vi "AK-LNI Befehl und Antwort_ALT.vi"(7 "Kanalnummer (0)":u8 max=99 step=1, 8 "Fehler (Eingang)":errorcluster, 9 "Sendedaten":string[](array[string]), 10 "Befehl (4 Zeichen)":string, 11 "VISA resource name":refnum<visa-resource-name>) -> (0 "Fehler (Ausgang)":errorcluster, 1 "ES (Error Status)":string, 2 "Empfangsdaten":string[](array[string]), 3 "VISA resource name out":refnum<visa-resource-name>, 4 "Daten":string, 5 "Befehl (Antwort)":string)   [LabVIEW 2020, in "Linearisierung v2.lvlib" / "Gasteiler.lvlib" / "AK Komm Gasteiler.lvlib" / "Alter Gasteiler.lvlib"]
doc: "Vollständige Gerätekommunikation für Inbetriebnahme und als Muster für spezielle Befehle. Sendet ein vollständiges Befehls-Telegramm und liefert die Geräteantwort als 1D-Array aus Strings \"Empfangsdaten\", in dem die einzelnen Argumente getrennt verfügbar sind.\n\n\"Befehl\": immer vier ASCII-Zeichen (Großbuchstaben)\n\n\"Daten\": 1D-Array aus ASCII-Strings nach Vorgabe des Befehls."
uses:
  Alter Gasteiler.lvlib
  AK Komm Gasteiler.lvlib
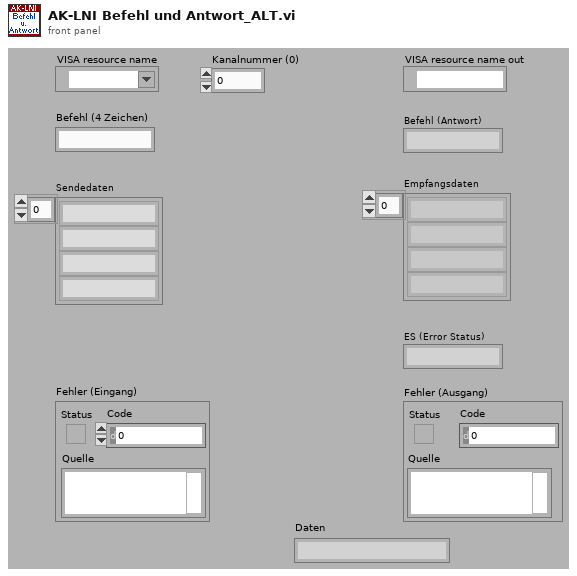
[diagram p1: front panel]
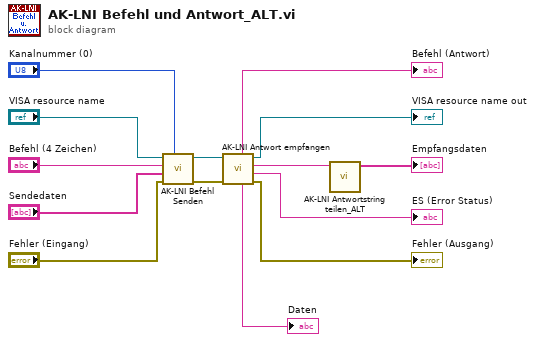
[diagram p0: block diagram]
diagram:
  n1 = call "AK-LNI Befehl Senden.vi"("Kanalnummer (K0)"="Kanalnummer (0)", "Fehler (Eingang)"="Fehler (Eingang)", "Daten"="Sendedaten", "Befehl (4 Zeichen)"="Befehl (4 Zeichen)", "VISA resource name"="VISA resource name") -> ("Fehler (Ausgang)"=w11:errorcluster, "VISA resource name out"=w13:refnum<visa-resource-name>)  [unwired: 5 in]
  n2 = call "AK-LNI Antwort empfangen.vi"("Fehler (Eingang)"=w11, "VISA resource name"=w13) -> ("Fehler (Ausgang)"=→"Fehler (Ausgang)":errorcluster, "ES (Error Status)"=→"ES (Error Status)":string, "Daten"=w4:string, "VISA resource name out"=→"VISA resource name out":refnum<visa-resource-name>, "Lesepuffer"=→"Daten":string, "Befehl"=→"Befehl (Antwort)":string)  [unwired: 4 in]
  n3 = call "AK-LNI Antwortstring teilen_ALT.vi"("Antwortstring"=w4) -> ("Empfangsdaten"=→"Empfangsdaten":string[])  [unwired: 10 in]
